vi "Reports.Results CSV Data to JSON File With Data Files.vi"(6 "File Data Objs":T1[](array[typedef]), 7 "Temp Folder":path, 8 "error in (no error)":errorcluster, 9 "CSV Data File":path, 10 "File Name":string, 11 "Folder":path) -> (0 "error out":errorcluster)   [LabVIEW 2018]
uses:
  Report.Result FileDataObject.ctl
  <vilib>/KATE/Files/File Utils.lvlib
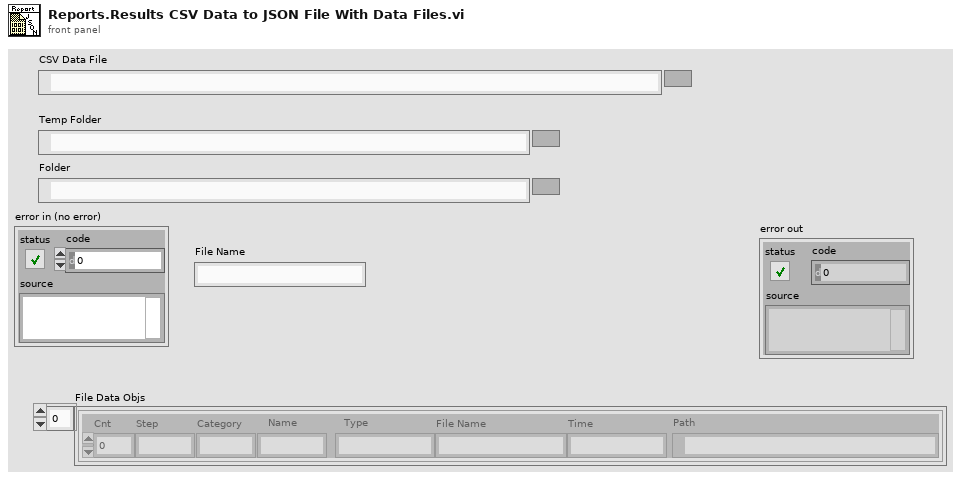
[diagram p1: front panel]
types:
  T1 = typedef "Report.Result FileDataObject.ctl" = cluster{"Cnt":i32, "Step":string, "Category":string, "Name":string, "Type":string, "File Name":string, "Time":string, "Path":path}
  T2 = typedef "Report.Result Data JSON V2.0.0.ctl" = cluster{"Type":string, "Version":string, "TestEvent":T3, "UUTInfo":T5, "Station":T6, "TestSequence":T7, "ResultData":T8[], "DataObjs":T9[]}
  T3 = typedef "Report.Result Test Event.ctl" = cluster{"ProcessStep":string, "StartTime":string, "EndTime":string, "Mode":string, "Operator":string, "Comment":string, "Result":T4}
  T4 = typedef "Report.Result State.ctl" = cluster{"State":string, "Code":i32, "Desc":string, "Details":string}
  T5 = typedef "Report.Result UUTInfo.ctl" = cluster{"Product":string, "Description":string, "PN":string, "SN":string, "LotNumber":string, "DateCode":string, "AltID":string, "Revision":string, "Properties":cluster{"Name":string, "Value":string}[]}
  T6 = typedef "Report.Result Test Station.ctl" = cluster{"Name":string, "Location":string, "ConfigID":string, "PCName":string, "Slot":string}
  T7 = typedef "Report.Result Test Sequence.ctl" = cluster{"Name":string, "Setup":cluster{"Name":string, "Value":string}[]}
  T8 = typedef "Report.Result Measurement JSON Safe.ctl" = cluster{"Cnt":i32, "Step":string, "Category":string, "Name":string, "Value":string, "Units":string, "LimType":string, "LL":string, "UL":string, "Time":string, "Result":T4}
  T9 = typedef "Report.Result DataObject.ctl" = cluster{"Cnt":i32, "Step":string, "Category":string, "Name":string, "Type":string, "FileName":string, "Time":string}
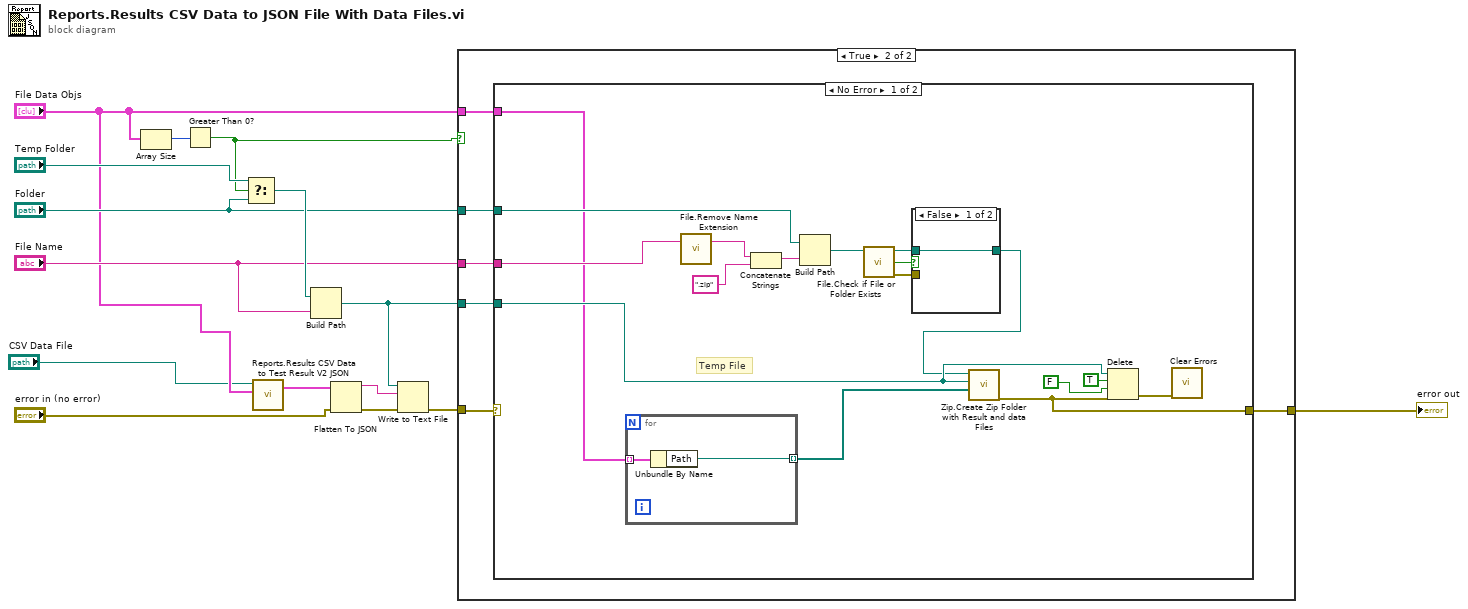
[diagram p0: block diagram]
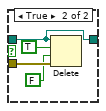
[diagram p3: hidden frame]
diagram:
  n1 = Array Size(array="File Data Objs") -> (size(s)=w11:i32)
  n2 = Greater Than 0?(x=w11) -> (x > 0?=w8:bool)
  n3 = Select(t="Temp Folder", s=w8, f="Folder") -> (s? t:f=w9:path)
  n4 = call "Reports.Results CSV Data to Test Result V2 JSON.vi"("File Data Objs"="File Data Objs", "CSV File"="CSV Data File") -> ("Test Result V2"=w14:T2)  [unwired: 3 in]
  n5 = Build Path(base path=w9, name or relative path="File Name") -> (appended path=w6:path)
  n6 = Flatten To JSON(anything=w14, error in (no error)="error in (no error)") -> (JSON string=w15:string, 11:w13:errorcluster)  [unwired: 1 in]
  n7 = Write to Text File(file (use dialog)=w6, text=w15, error in=w13) -> (error out=w7:errorcluster)  [unwired: 1 in, 2 out]
  n8 = case shown="True" w8 {
    tunnel: w7 -> [w16 w22]
    tunnel: w6 -> [_ w17]
    tunnel: [w16 w21] -> w5
    tunnel: "File Name" -> [_ w20]
    tunnel: "Folder" -> [_ w19]
    tunnel: "File Data Objs" -> [_ w18]
    frame False {
      # "Done\nOnly Write JSON file"
    }
    frame True {
      n9 = case shown="No Error" w22 {
        selector: w22 -> [_ w47]
        tunnel: [w31 w47] -> w21
        tunnel: w20 -> [w34 _]
        tunnel: w19 -> [w33 _]
        tunnel: w18 -> [w29 _]
        tunnel: w17 -> [w32 _]
        frame No Error {
          # "Temp File"
          n10 = for {
            tunnel: w29 -> [w46] mode=indexing
            tunnel: [w45] -> w28 mode=indexing
            n11 = Unbundle By Name(w46) -> ("Path"=w45:path)
          }
          n12 = call <vilib>:"File.Remove Name Extension.vi"("File Name"=w34) -> ("Name Less Ext"=w38:string)  [unwired: 1 in, 1 out]
          n13 = Concatenate Strings(w38, ".zip" ("string")) -> (w39:string)
          n14 = Build Path(base path=w33, name or relative path=w39) -> (appended path=w24:path)
          n15 = call <vilib>:"File.Check if File or Folder Exists.vi"("Path"=w24) -> ("error out"=w27:errorcluster, "Exists"=w25:bool, "Dup Path"=w26:path)  [unwired: 6 in, 2 out]
          n16 = case shown="False" w25 {
            tunnel: w27 -> [_ w44]
            tunnel: w26 -> [w40 w41]
            tunnel: [w40 w41] -> w23
            frame False {
            }
            frame True {
              n17 = Delete(path (use dialog)=w41, entire hierarchy (F)=TRUE, confirm (F)=FALSE, error in=w44) -> ()  [unwired: 1 in, 3 out]
            }
          }
          n18 = call "Zip.Create Zip Folder with Result and data Files.vi"("Data Files"=w28, "Result File"=w32, "Output Zip File"=w23) -> ("error out"=w31:errorcluster)  [unwired: 8 in]
          n19 = Delete(path (use dialog)=w32, entire hierarchy (F)=TRUE, confirm (F)=FALSE, error in=w31) -> (error out=w30:errorcluster)  [unwired: 1 in, 2 out]
          n20 = call <vilib>:"Clear Errors.vi"("error in (no error)"=w30) -> ()  [unwired: 5 in, 2 out]
        }
        frame Error {
        }
      }
    }
  }
  "error out" <- w5
